vi "ConfigureClient.vi"(8 "error in (no error)":errorcluster, 10 "Start OPC Client":bool, 11 "config in":T1) -> (0 "error out":errorcluster, 3 "config out":T1)   [LabVIEW 2017, in "OPCUAClient.lvlib"]
uses:
  <vilib>/addons/InsightCM/Devices/Shared/Common/OPCUAClient/OPCUAClient.lvlib
  <vilib>/addons/InsightCM/Devices/Shared/Common/OPCUAClient/controls/config.ctl
  <vilib>/OPCUA/controls/OPC UA Client Refnum.ctl
  <vilib>/addons/InsightCM/Devices/Shared/Common/OPCUAClient/controls/group.ctl
  <vilib>/addons/InsightCM/Devices/Shared/Common/OPCUAClient/controls/tag.ctl
  <vilib>/addons/InsightCM/Utilities/GlobalConfiguration/GlobalConfiguration.lvlib
  <vilib>/addons/InsightCM/Utilities/PropertyHelpers/PropertyHelpers.lvlib
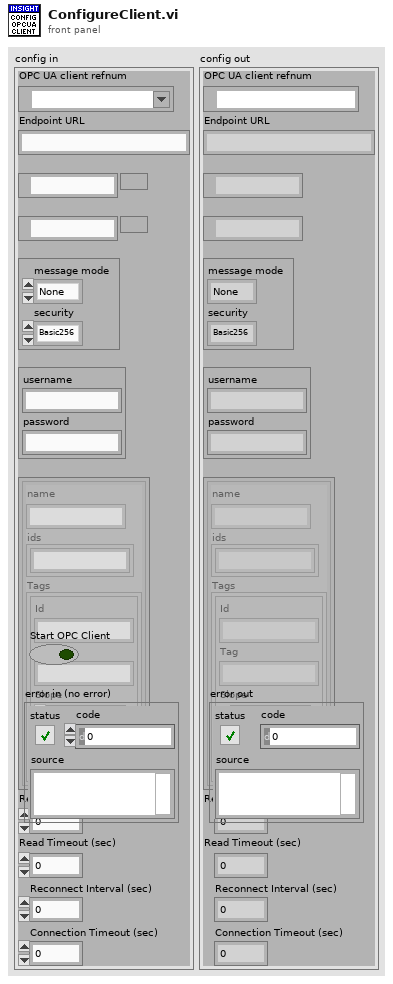
[diagram p1: front panel]
types:
  T1 = typedef "OPCUAClient.lvlib/config.ctl" = cluster{"OPC UA client refnum":T2, "Endpoint URL":string, "Client Certificate":path, "Server Certificate":path, "security policy":cluster{"message mode":enum16{"None", "Sign", "Sign and Encrypt"}, "security":enum16{"Basic256", "Basic128Rsa15"}}, "username/password":cluster{"username":string, "password":string}, "groups":T3[], "Read Interval (sec)":dbl, "Read Timeout (sec)":dbl, "Reconnect Interval (sec)":dbl, "Connection Timeout (sec)":dbl}
  T2 = typedef "OPC UA Client Refnum.ctl" = refnum<k21>
  T3 = typedef "OPCUAClient.lvlib/group.ctl" = cluster{"name":string, "ids":string[], "Tags":T4[]}
  T4 = typedef "OPCUAClient.lvlib/tag.ctl" = cluster{"Id":string, "Tag":string, "Slope":dbl, "Offset":dbl}
  T5 = typedef "DataSource.ctl" = cluster{"Id":string, "Type":string, "Name":string, "MeasType":string, "Properties":T6[]}
  T6 = typedef "KeyValuePair.ctl" = cluster{"Key":string, "Value":string}
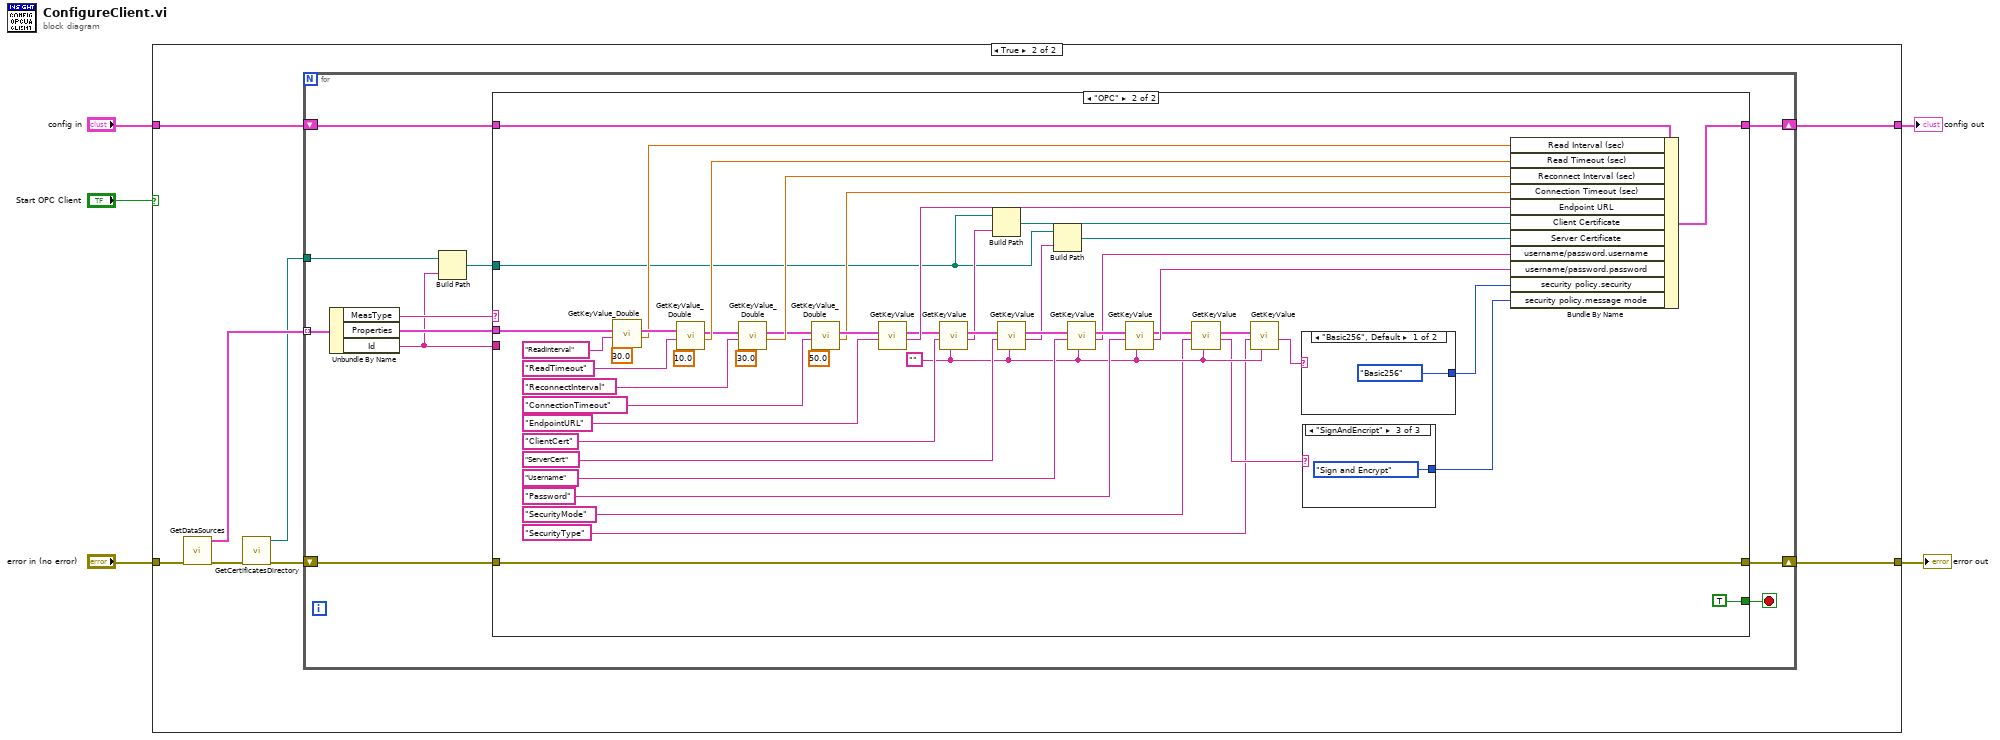
[diagram p0: block diagram]
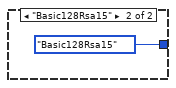
[diagram p4: hidden frame]
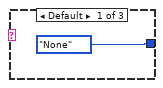
[diagram p5: hidden frame]
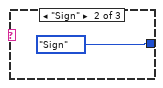
[diagram p6: hidden frame]
diagram:
  n1 = case shown="True" "Start OPC Client" {
    tunnel: "error in (no error)" -> [w7 w12]
    tunnel: [w7 w15] -> w3
    tunnel: [w6 w13] -> w2
    tunnel: "config in" -> [w6 w14]
    frame False {
    }
    frame True {
      n2 = call <vilib>:"GetDataSources.vi"("error in (no error)"=w12) -> ("error out"=w10:errorcluster, "data sources"=w11:T5[])  [unwired: 8 in, 1 out]
      n3 = call <vilib>:"GetCertificatesDirectory.vi"("error in (no error)"=w10) -> ("error out"=w9:errorcluster, "application directory"=w8:path)  [unwired: 9 in]
      n4 = for {
        shift-right: [w24] -> w13
        shift-left: w14 -> [w25]
        shift-right: [w26] -> w15
        shift-left: w9 -> [w23]
        tunnel: w11 -> [w22] mode=indexing
        tunnel: w8 -> [w18]
        stop <- w20 stop-if-true
        n5 = Unbundle By Name(w22) -> ("MeasType"=w21:string, "Properties"=w19:T6[], "Id"=w17:string)
        n6 = Build Path(base path=w18, name or relative path=w17) -> (appended path=w16:path)
        n7 = case shown="\"OPC\"" w21 {
          tunnel: [w27 w60] -> w26
          tunnel: w25 -> [w28 w75]
          tunnel: [w28 w74] -> w24
          tunnel: w23 -> [w27 w60]
          tunnel: [_ TRUE] -> w20
          tunnel: w19 -> [_ w72]
          tunnel: w17 -> [_ _]
          tunnel: w16 -> [_ w31]
          frame Default {
          }
          frame "OPC" {
            w40 = ""
            n8 = call <vilib>:"GetKeyValue_Double.vi"("default"=30.0, "key"="ReadInterval", "key value pairs"=w72) -> ("value"=w67:dbl, "key value pairs out"=w71:T6[])  [unwired: 6 in, 1 out]
            n9 = call <vilib>:"GetKeyValue_Double.vi"("default"=10.0, "key"="ReadTimeout", "key value pairs"=w71) -> ("value"=w65:dbl, "key value pairs out"=w59:T6[])  [unwired: 6 in, 1 out]
            n10 = call <vilib>:"GetKeyValue_Double.vi"("default"=30.0, "key"="ReconnectInterval", "key value pairs"=w59) -> ("value"=w61:dbl, "key value pairs out"=w55:T6[])  [unwired: 6 in, 1 out]
            n11 = call <vilib>:"GetKeyValue_Double.vi"("default"=50.0, "key"="ConnectionTimeout", "key value pairs"=w55) -> ("value"=w53:dbl, "key value pairs out"=w56:T6[])  [unwired: 6 in, 1 out]
            n12 = call <vilib>:"GetKeyValue.vi"("key"="EndpointURL", "key value pairs"=w56) -> ("value"=w58:string, "key value pairs out"=w52:T6[])  [unwired: 7 in, 1 out]
            n13 = call <vilib>:"GetKeyValue.vi"("default value"=w40, "key"="ClientCert", "key value pairs"=w52) -> ("value"=w33:string, "key value pairs out"=w51:T6[])  [unwired: 6 in, 1 out]
            n14 = Build Path(base path=w31, name or relative path=w33) -> (appended path=w32:path)
            n15 = call <vilib>:"GetKeyValue.vi"("default value"=w40, "key"="ServerCert", "key value pairs"=w51) -> ("value"=w30:string, "key value pairs out"=w47:T6[])  [unwired: 6 in, 1 out]
            n16 = Build Path(base path=w31, name or relative path=w30) -> (appended path=w29:path)
            n17 = call <vilib>:"GetKeyValue.vi"("default value"=w40, "key"="Username", "key value pairs"=w47) -> ("value"=w44:string, "key value pairs out"=w48:T6[])  [unwired: 6 in, 1 out]
            n18 = call <vilib>:"GetKeyValue.vi"("default value"=w40, "key"="Password", "key value pairs"=w48) -> ("value"=w43:string, "key value pairs out"=w41:T6[])  [unwired: 6 in, 1 out]
            n19 = call <vilib>:"GetKeyValue.vi"("default value"=w40, "key"="SecurityMode", "key value pairs"=w41) -> ("value"=w38:string, "key value pairs out"=w42:T6[])  [unwired: 6 in, 1 out]
            n20 = call <vilib>:"GetKeyValue.vi"("default value"=w40, "key"="SecurityType", "key value pairs"=w42) -> ("value"=w37:string)  [unwired: 6 in, 2 out]
            n21 = case shown="\"Basic256\", Default" w37 {
              tunnel: [enum16{"Basic256", "Basic128Rsa15"}."Basic256" ("security") enum16{"Basic256", "Basic128Rsa15"}."Basic128Rsa15" ("security")] -> w36
              frame "Basic256", Default {
              }
              frame "Basic128Rsa15" {
              }
            }
            n22 = case shown="\"SignAndEncript\"" w38 {
              tunnel: [enum16{"None", "Sign", "Sign and Encrypt"}."None" ("message mode") enum16{"None", "Sign", "Sign and Encrypt"}."Sign" ("message mode") enum16{"None", "Sign", "Sign and Encrypt"}."Sign and Encrypt" ("message mode")] -> w35
              frame Default {
              }
              frame "Sign" {
              }
              frame "SignAndEncript" {
              }
            }
            n23 = Bundle By Name(cluster=w75, "Read Interval (sec)"=w67, "Read Timeout (sec)"=w65, "Reconnect Interval (sec)"=w61, "Connection Timeout (sec)"=w53, "Endpoint URL"=w58, "Client Certificate"=w32, "Server Certificate"=w29, "username/password.username"=w44, "username/password.password"=w43, "security policy.security"=w36, "security policy.message mode"=w35) -> (w74:T1)
          }
        }
      }
    }
  }
  "config out" <- w2
  "error out" <- w3
